vi "miclose.vi"(1 "错误输入（无错误）":errorcluster, 2 "连接ID":refnum<k5>) -> (0 "错误输出":errorcluster)   [LabVIEW 2017]
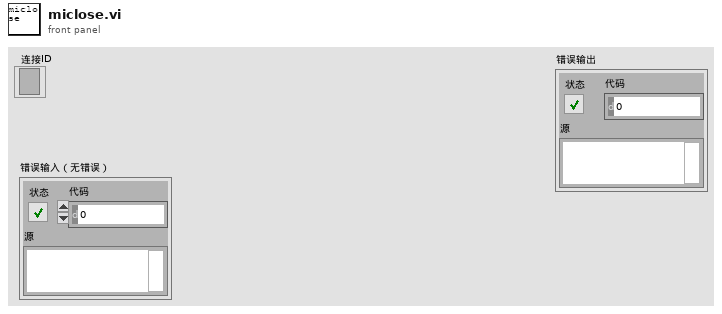
[diagram p1: front panel]
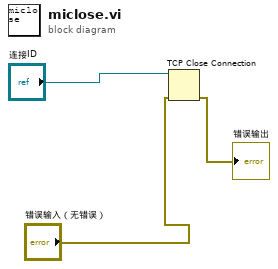
[diagram p0: block diagram]
diagram:
  n1 = TCP Close Connection(connection ID="连接ID", error in (no error)="错误输入（无错误）") -> (error out=→"错误输出":errorcluster)  [unwired: 1 in, 1 out]
